vi "Draw Button by Index and State.vi"(6 "Force redraw ?":bool, 8 "error in (no error)":errorcluster, 9 "index":i32, 10 "Button State":T3, 11 "State":T1={"Buttons Displayed"=0, "Button States"=[], "Button Size"=0, "Button Style"=enum."Classic", "Active Button"=0, "Force Regen?"=FALSE, "Tip String Ref"=refnum}) -> (0 "error out":errorcluster, 1 "Image (no button)":picture, 2 "Picture Out":picture, 3 "State out":T1={"Buttons Displayed"=0, "Button States"=[], "Button Size"=0, "Button Style"=enum."Classic", "Active Button"=0, "Force Regen?"=FALSE, "Tip String Ref"=refnum} caption="State")   [LabVIEW 2012, in "Toolbar.xctl"]
doc: "Utility method to draw a button in a particular state. Looks up the button class instance and calls that to generate the button image, using the current button size and style."
uses:
  Toolbar.xctl
  Button_Class/Type Defs/Button Status.ctl
  Toolbar State.ctl
  Button_Class/Button.lvclass
  Button_Class/Type Defs/Button Style.ctl
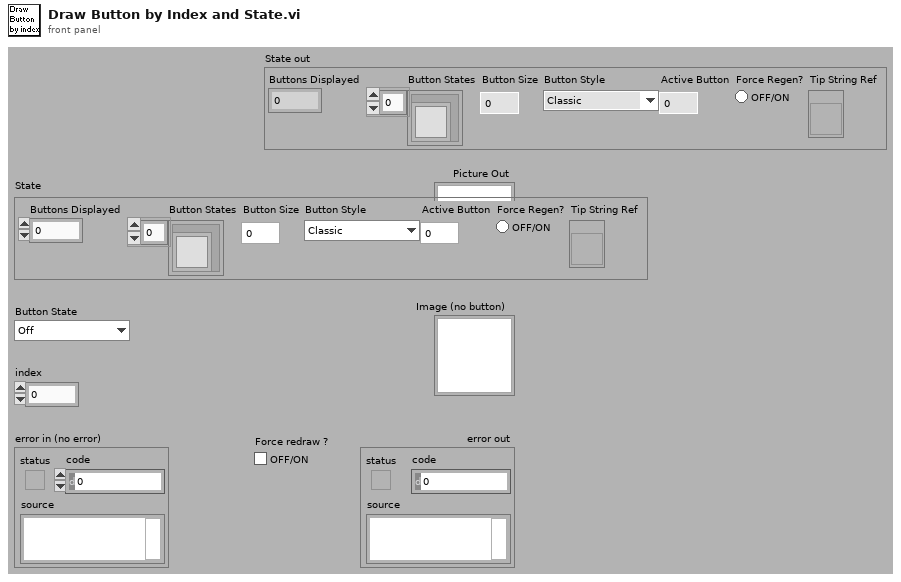
[diagram p1: front panel]
types:
  T1 = typedef "Toolbar.xctl/Toolbar State.ctl" = cluster{"Buttons Displayed":i32, "Button States":refnum<class "Button.lvclass">[], "Button Size":i32, "Button Style":T2, "Active Button":i32, "Force Regen?":bool, "Tip String Ref":refnum<vi>}
  T2 = typedef "Button.lvclass/Button Style.ctl" = enum16{"System", "Modern", "Classic", "Rounded", "Silver", "Ni Theme", "Metallic"}
  T3 = typedef "Button.lvclass/Button Status.ctl" = enum16{"Off", "Hover", "On", "Disabled"}
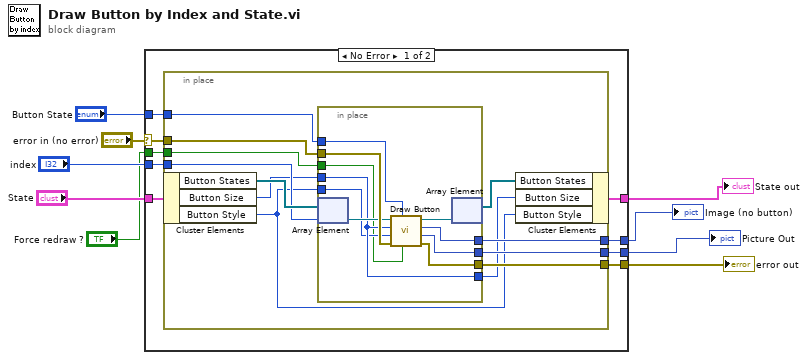
[diagram p0: block diagram]
diagram:
  n1 = case shown="No Error" "error in (no error)" {
    selector: "error in (no error)" -> [w14 w42]
    tunnel: "Button State" -> [w17 _]
    tunnel: "index" -> [w18 _]
    tunnel: [w13 _] -> w1
    tunnel: [w15 w42] -> w7
    tunnel: "State" -> [w12 w41]
    tunnel: [w16 _] -> w2
    tunnel: "Force redraw ?" -> [w11 _]
    tunnel: [w10 w41] -> w3
    frame No Error {
      n2 = in-place {
        in-place-border: w18 -> [w24]
        in-place-border: w17 -> [w30]
        in-place-border: [w29] -> w16
        in-place-border: [w28] -> w15
        in-place-border: w14 -> [w27]
        in-place-border: [w26] -> w13
        in-place-border: w11 -> [w19]
        n3 = in-place-cluster #1(w12) -> ("Button States"=w25:refnum<class "Button.lvclass">[], "Button Size"=w22:i32, "Button Style"=w20:T2)
        n4 = in-place {
          in-place-border: w30 -> [w40]
          in-place-border: [w39] -> w29
          in-place-border: [w38] -> w28
          in-place-border: w27 -> [w37]
          in-place-border: [w36] -> w26
          in-place-border: w22 -> [w33]
          in-place-border: [w33] -> w21
          in-place-border: w20 -> [w32]
          in-place-border: w19 -> [w31]
          n5 = in-place-array #2(w25, w24) -> (w35:refnum<class "Button.lvclass">)
          n6 = call "Draw Button.vi"("Force redraw ?"=w31, "Button State"=w40, "error in (no error)"=w37, "Button Style"=w32, "Button Size"=w33, "Button.lvclass"=w35) -> ("error out"=w38:errorcluster, "Picture Out"=w36:picture, "Image (no button)"=w39:picture, "Button.lvclass Out"=w34:refnum<class "Button.lvclass">)  [unwired: 2 out]
          n7 = in-place-array #2(w34) -> (w23:refnum<class "Button.lvclass">[])  [unwired: 1 out]
        }
        n8 = in-place-cluster #1("Button States"=w23, "Button Size"=w21, "Button Style"=w20) -> (w10:T1)
      }
    }
    frame Error {
    }
  }
  "Picture Out" <- w1
  "error out" <- w7
  "Image (no button)" <- w2
  "State out" <- w3
